vi "fetchBTFData_mc_1.1.vi"(0 "Funcion":u16(ring) items=["Init", "Run", "Close"], 1 "Port (Deprecated)":u16=10000) -> (3 "lastTrigger":i32, 4 "Array":i32[](array[numeric]), 6 "ReadError":bool, 7 "DataReady":bool)   [LabVIEW 2014]
panel:
  # "Version:\n- 1.0 UDP to MC\n- 1.1 deduce dataready \n\nto be done:\n- manage errori"
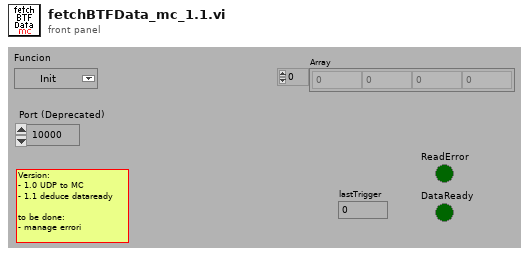
[diagram p1: front panel]
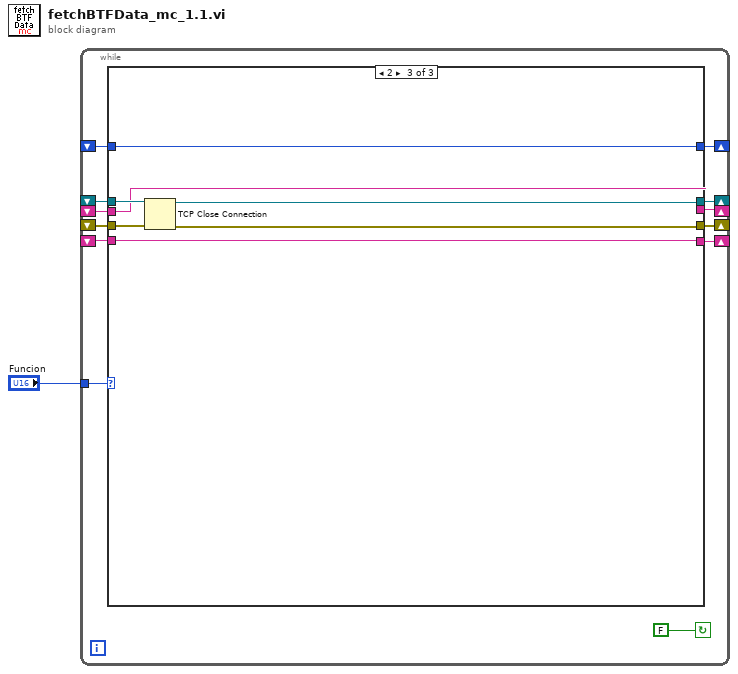
[diagram p0: block diagram]
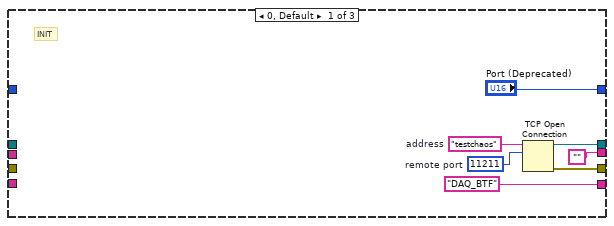
[diagram p2: hidden frame]
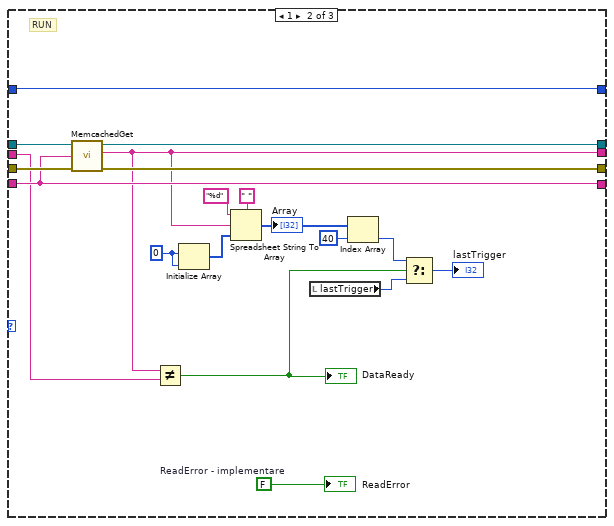
[diagram p3: hidden frame]
diagram:
  n1 = while {
    shift-left: _ -> [w12]
    shift-right: [w11] -> _
    tunnel: "Funcion" -> [w13]
    shift-right: [w9] -> _
    shift-left: _ -> [w7]
    shift-right: [w8] -> _
    shift-left: _ -> [w6]
    shift-right: [w5] -> _
    shift-left: _ -> [w4]
    shift-right: [w3] -> _
    shift-left: _ -> [w2]
    stop <- FALSE continue-if-true
    n2 = case shown="2" w13 {
      tunnel: w12 -> [_ w39 w42]
      tunnel: ["Port (Deprecated)" w39 w42] -> w11
      tunnel: [w17 w27 w44] -> w9
      tunnel: [w16 w26 w43] -> w8
      tunnel: w7 -> [_ w29 w46]
      tunnel: w6 -> [_ w28 w45]
      tunnel: ["DAQ_BTF" w25 w41] -> w5
      tunnel: w4 -> [_ w25 w41]
      tunnel: ["" w24 w40] -> w3
      tunnel: w2 -> [_ w23 w40]
      frame 0, Default {
        w18 = u16 11211  # remote port
        w19 = "testchaos"  # address
        # "INIT"
        n3 = TCP Open Connection(address=w19, remote port or service name=w18) -> (connection ID=w17:refnum<k5>, error out=w16:errorcluster)  [unwired: 3 in]
      }
      frame 1 {
        w21 = FALSE  # ReadError - implementare
        w33 = 0
        # "RUN"
        n4 = call "MemcachedGet.vi"("connection ID"=w29, "key"=w25, "error in (no error)"=w28) -> ("connection ID out"=w27:refnum<k5>, "data out"=w24:string, "error out"=w26:errorcluster)  [unwired: 1 out]
        n5 = Not Equal?(x=w24, y=w23) -> (x != y?=w22:bool)
        "DataReady" <- w22
        n6 = Initialize Array(w33, w33) -> (w34:i32[])
        n7 = Spreadsheet String To Array(delimiter (Tab)=" ", format string="%d", spreadsheet string=w24, array type (2D Dbl)=w34) -> (array=w30:i32[])
        "Array" <- w30
        n8 = local read "lastTrigger"() -> (w35:i32)
        n9 = Index Array(array=w30, index=40) -> (element=w37:i32)
        n10 = Select(t=w37, s=w22, f=w35) -> (s? t:f=→"lastTrigger":i32)
        "ReadError" <- w21
      }
      frame 2 {
        n11 = TCP Close Connection(connection ID=w46, error in (no error)=w45) -> (connection ID out=w44:refnum<k5>, error out=w43:errorcluster)  [unwired: 1 in]
      }
    }
  }
